vi "Multiple Chassis Synchronization - Scopes Synchronized without TCLK.vi"() -> ()   [LabVIEW 2026]
uses:
  SubVIs/NI SYNC Abstraction/Lib/Clock Routing.ctl
  <instrlib>/niScope/Controls/niScope export destinations.ctl
  SubVIs/NI SYNC Abstraction/Lib/Trigger Routing.ctl
  Types/State.WithoutTclk.ctl
  <instrlib>/niScope/Controls/niScope input clock source.ctl
  Types/MyVariables.ctl
  <instrlib>/niScope/Controls/niScope exportable signals.ctl
  <instrlib>/niFgen/niFgen.llb/niFgen Output Mode.ctl
  <instrlib>/niScope/Configure/Trigger/niScope Configure Trigger Edge.vi
  <instrlib>/niScope/Configure/Trigger/niScope Configure Trigger Digital.vi
  SubVIs/NI SYNC Abstraction/Lib/Connect Clock Terminals-Array.vi
  SubVIs/NI SYNC Abstraction/Lib/Connect Clock Terminals.vi
  SubVIs/NI SYNC Abstraction/Lib/Connect Trigger Terminals.vi
  <instrlib>/niScope/Acquire/Fetch/niScope Fetch Cluster.vi
  SubVIs/NI SYNC Abstraction/Lib/Disonnect Trigger Terminals.vi
  SubVIs/NI SYNC Abstraction/Lib/Disconnect Clock Terminals-Array.vi
  SubVIs/NI SYNC Abstraction/Lib/Disconnect Clock Terminals.vi
  <instrlib>/niSync/niSync.llb/niSync Initialize (IVI).vi
panel:
  in  "Tab Control":T1(tab)
  in  "Master.Scope":refnum<k15>="PXI1_SCOPE1"
  in  "Rest.Scopes":refnum<k15>[](array[refnum])=["PXI2_SCOPE2"]
  in  "Master.6674T_1":refnum<k15>="PXI1_MasterSync"
  in  "Rest.6674T_1":refnum<k15>="PXI2_SlaveSync"
  in  "FGEN.Ref":refnum<k15>="PXI1_FGEN1"
  in  "Routing":enum32{"Clock Routing", "Reference Trigger"}(tab)
  in  "Rest.In --> Clk10":T2={"Source Terminal"="ClkIn", "Destination Terminal"="PXI_Clk10_In"}
  in  "Master.In --> Clk10":T2={"Source Terminal"="ClkIn", "Destination Terminal"="PXI_Clk10_In"}
  in  "Master.Clock --> Out":T2={"Source Terminal"="Oscillator", "Destination Terminal"="ClkOut"}
  in  "Rest.Ref Trigger Source":T3="VAL_RTSI_0"
  in  "Rest.PFI --> Ref Trigger":T4={"Source"="PFI0", "Destination"="PXI_Trig0", "Synchronization Clock"="SyncClkAsync"}
  in  "Master.Ref Trigger --> PFI":T4={"Source"="PXI_Trig0", "Destination"="PFI0", "Synchronization Clock"="SyncClkAsync"}
  in  "Master.Ref Trigger Export":T3="VAL_RTSI_0"
  out "Waveform Graph":T5(graph)
  out "Sample Offset":dbl
  out "error out":errorcluster
  out "Offset Time (s)":dbl format="%#_p"
  # "Scope"
  # "Sync"
  # "Master"
  # "Ref Trigger Export"
  # "None"
  # "None"
  # "None"
  # "Sync"
  # "Scope"
  # "Rest"
  # "Ref Trigger Source"
  # "None"
  # "None"
  # "None"
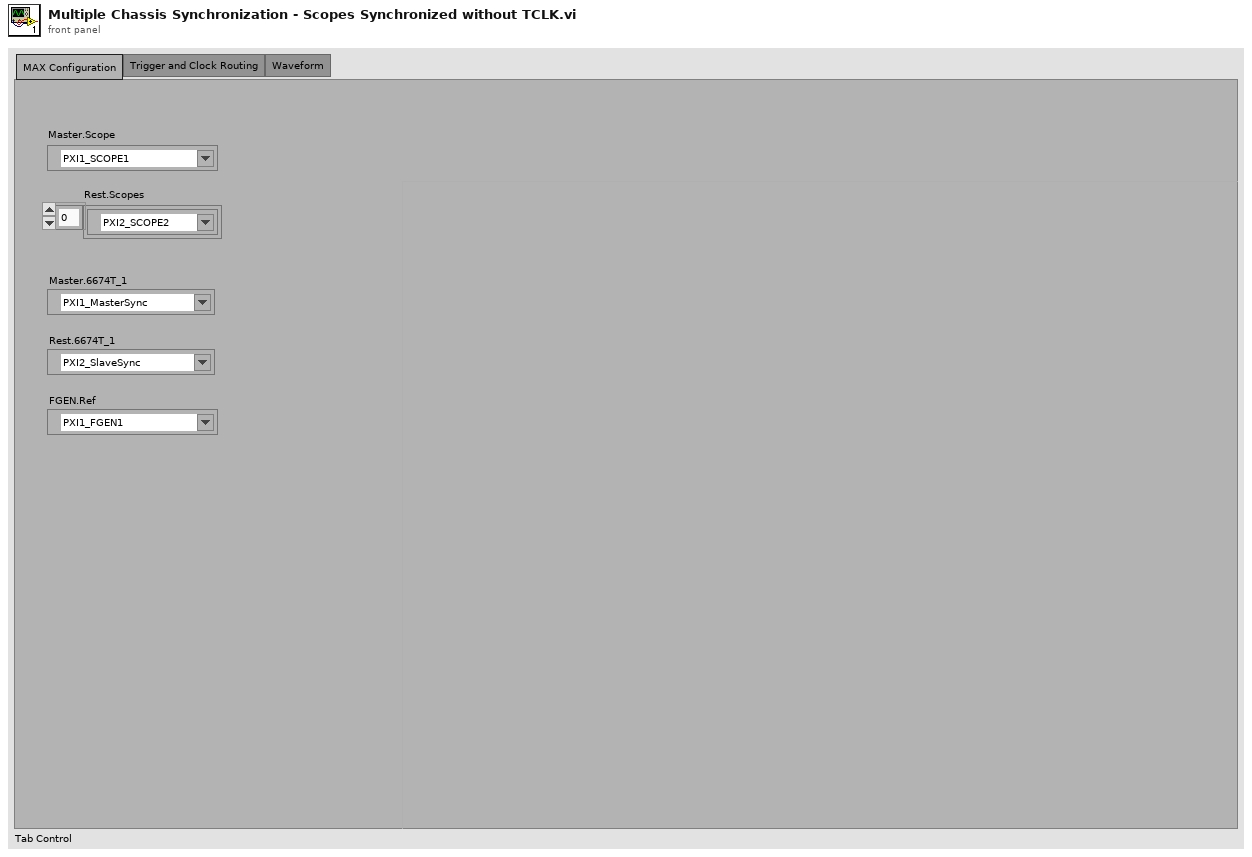
[diagram p1: front panel]
types:
  T1 = enum32{"MAX Configuration", "Trigger and Clock Routing", "Waveform"}
  T2 = typedef "Clock Routing.ctl" = cluster{"Source Terminal":string, "Destination Terminal":string}
  T3 = typedef "niScope export destinations.ctl" = string
  T4 = typedef "Trigger Routing.ctl" = cluster{"Source":string, "Destination":string, "Synchronization Clock":string}
  T5 = cluster{"relativeInitialX":dbl, "xIncrement":dbl, "wfm":dbl[]}[]
  T6 = typedef "niScope input clock source.ctl" = u16
  T7 = typedef "State.WithoutTclk.ctl" = enum16{"Initialize", "SCOPE: Config.Master", "SCOPE: Config.Rest", "SYNC: Device.Init", "SYNC: ConnectClock.Master", "SYNC: ConnectClock.Rest", "SYNC: ConnectRefTrigger.Master", "SYNC: ConnectRefTrigger.Rest", "SCOPE: Start", "FGEN: StartSquareWave", "SCOPE: Acquire", "FGEN: StopSquareWave", "SYNC: DisconnectRefTrigger.Master", "SYNC: DisconnectRefTrigger.Rest", "SYNC: DisconnectClock.Master", "SYNC: DisconnectClock.Rest", "Shutdown"}
  T8 = typedef "MyVariables.ctl" = cluster{"Master":cluster{"TimeSync.Ref":refnum<k15>, "TCLK.Ref":refnum<k20>, "Clock":cluster{"Clock --> Out":T2, "In --> Clk10":T2}, "Sync Pulse":cluster{"Sync Pulse Export":string, "Sync Pulse Export --> PFI":T4, "PFI --> Sync Pulse Source":T4, "Sync Pulse Source":string}, "Start Trigger":cluster{"Start Trigger Export":T3, "Start Trigger --> PFI":T4}, "Scope.Ref":refnum<k15>, "Ref Trigger":cluster{"Ref Trigger Export":T3, "Ref Trigger --> PFI":T4}}, "Rest":cluster{"TimeSync.Ref":refnum<k15>, "TCLK.Refs":refnum<k20>[], "Clock":cluster{"In --> Clk10":T2}, "Sync Pulse":cluster{"PFI --> Sync Pulse Source":T4, "Sync Pulse Source":string}, "Start Trigger":cluster{"PFI --> Start Trigger":T4, "Start Trigger Source":T3}, "Scope.Refs":refnum<k15>[], "Ref Trigger":cluster{"PFI --> Ref Trigger":T4, "Ref Trigger Source":T3}}, "FGEN.Ref":refnum<k15>}
  T9 = typedef "niScope exportable signals.ctl" = u16
  T10 = typedef "niFgen Output Mode.ctl" = u32
  T11 = cluster{"relativeInitialX":dbl, "xIncrement":dbl, "wfm":dbl[]}
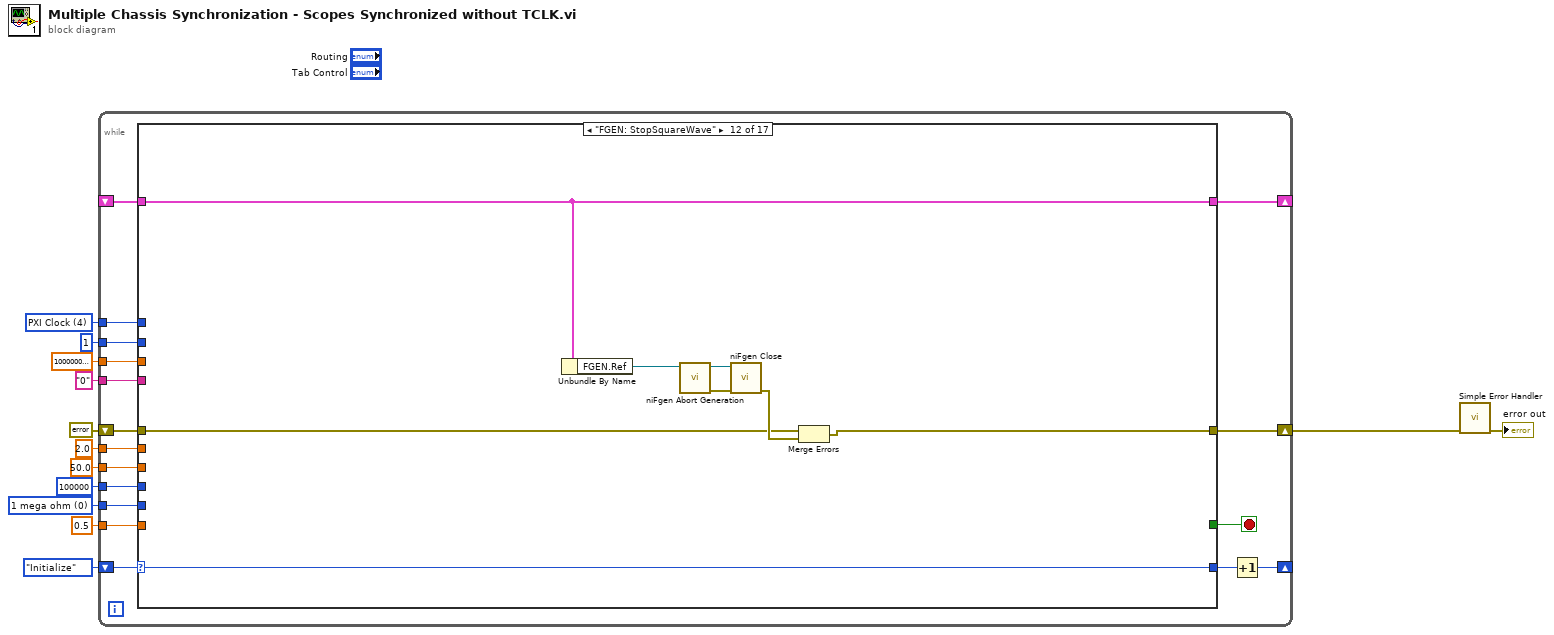
[diagram p0: block diagram]
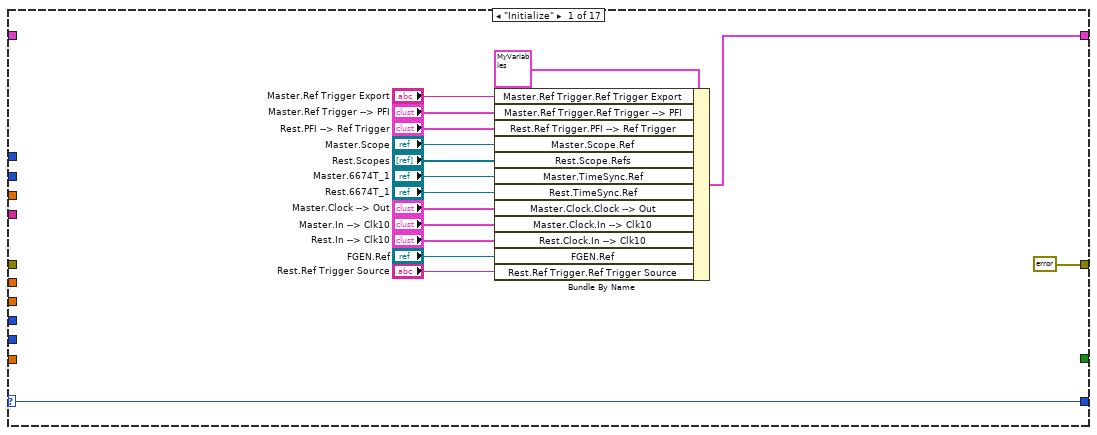
[diagram p2: hidden frame]
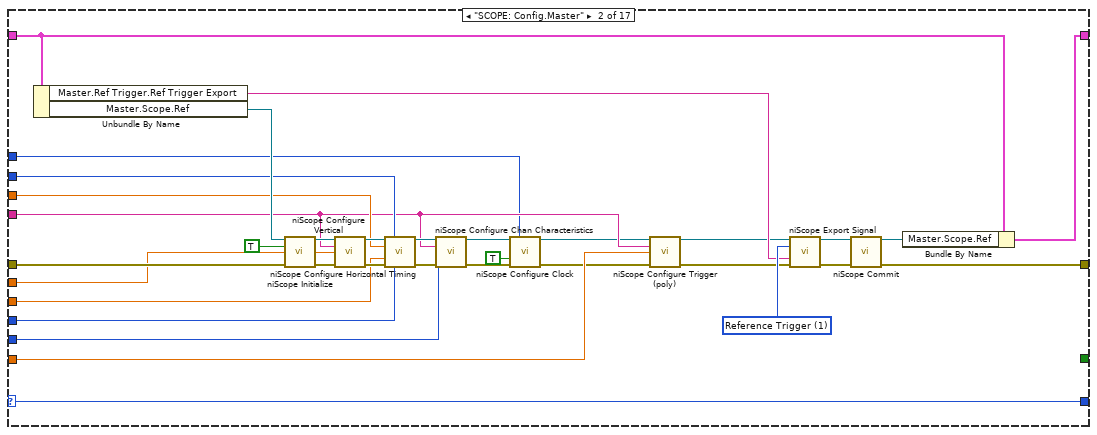
[diagram p3: hidden frame]
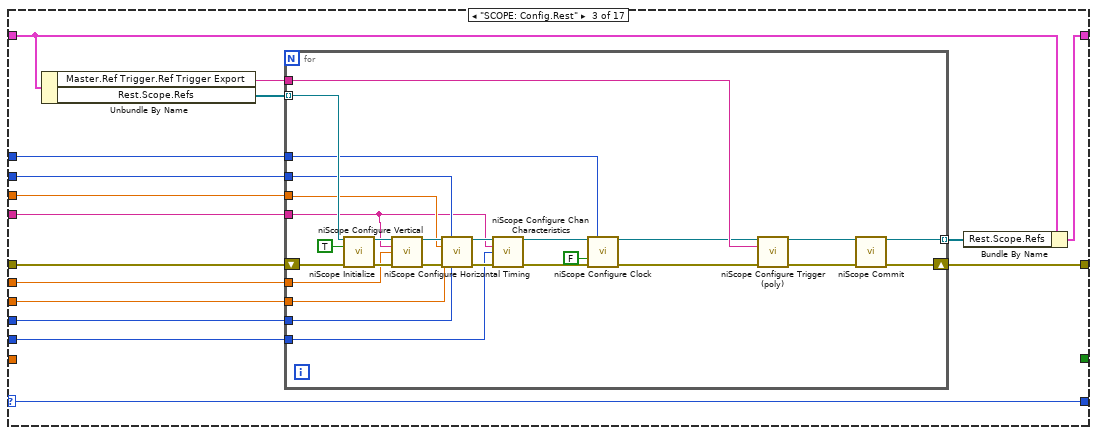
[diagram p4: hidden frame]
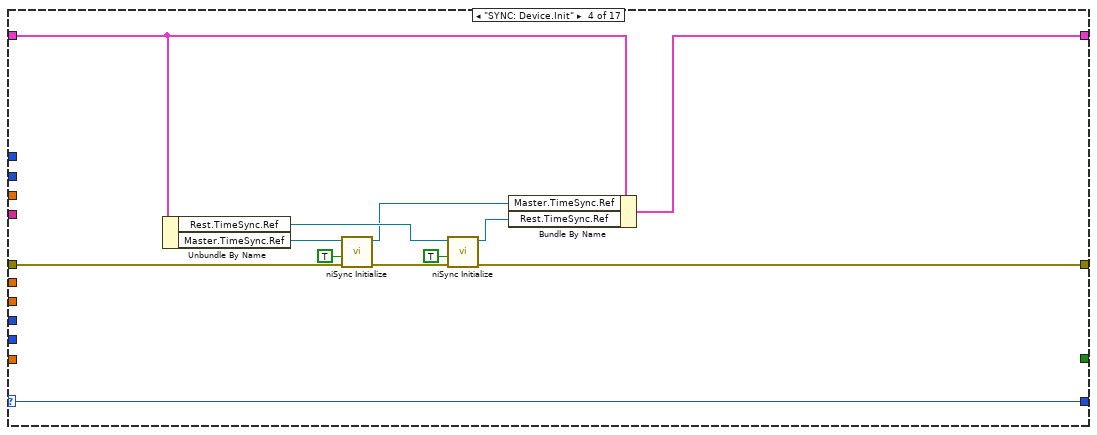
[diagram p5: hidden frame]
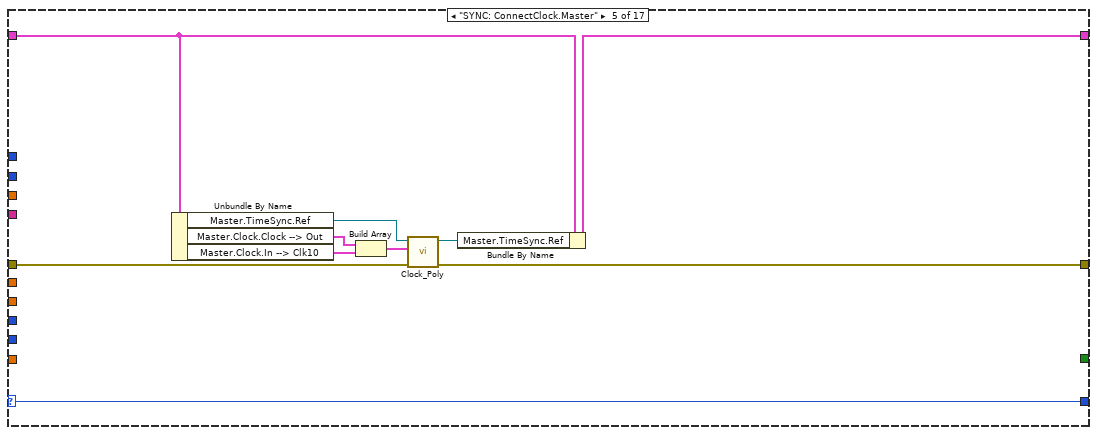
[diagram p6: hidden frame]
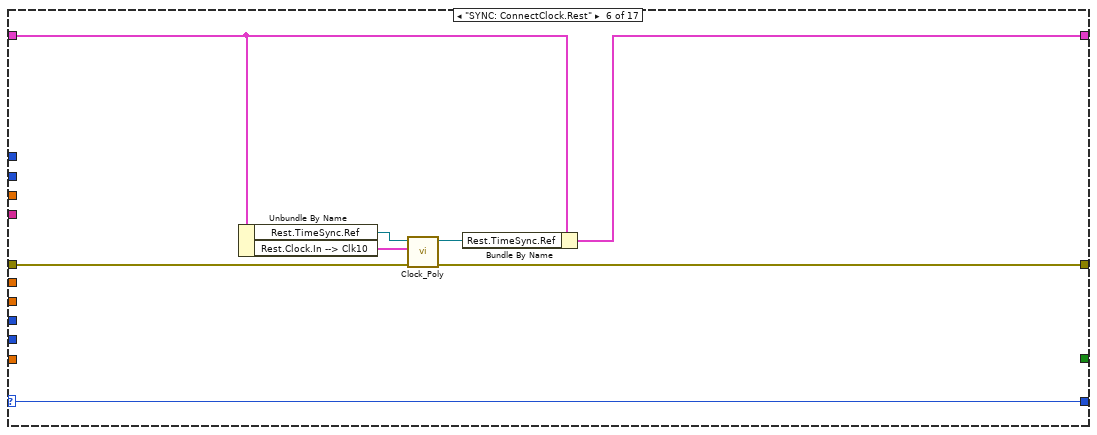
[diagram p7: hidden frame]
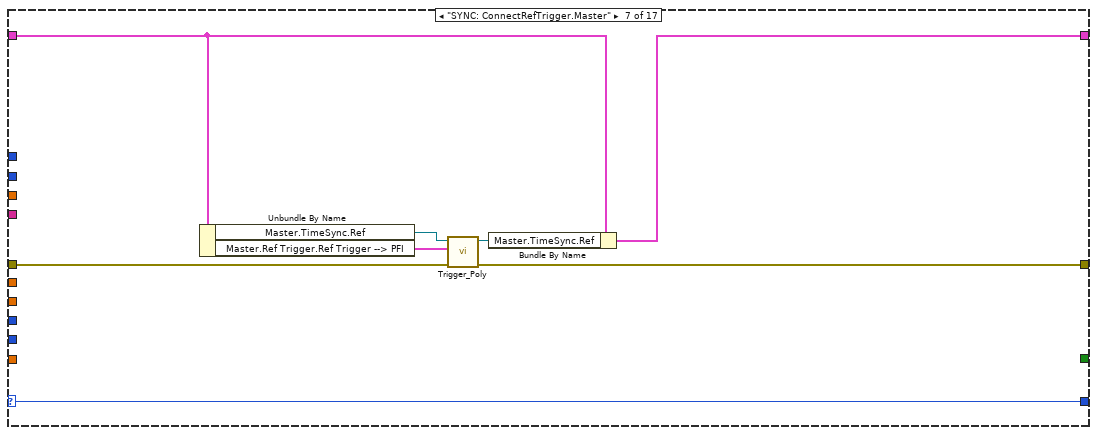
[diagram p8: hidden frame]
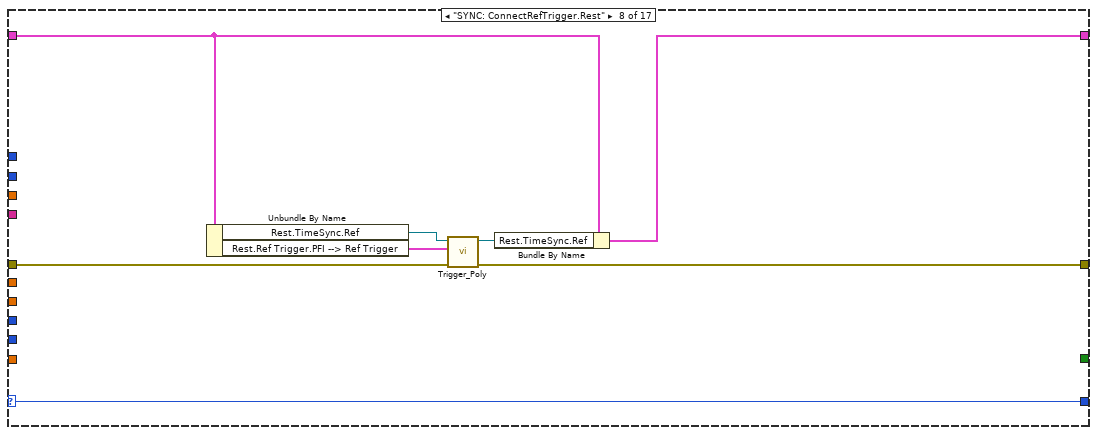
[diagram p9: hidden frame]
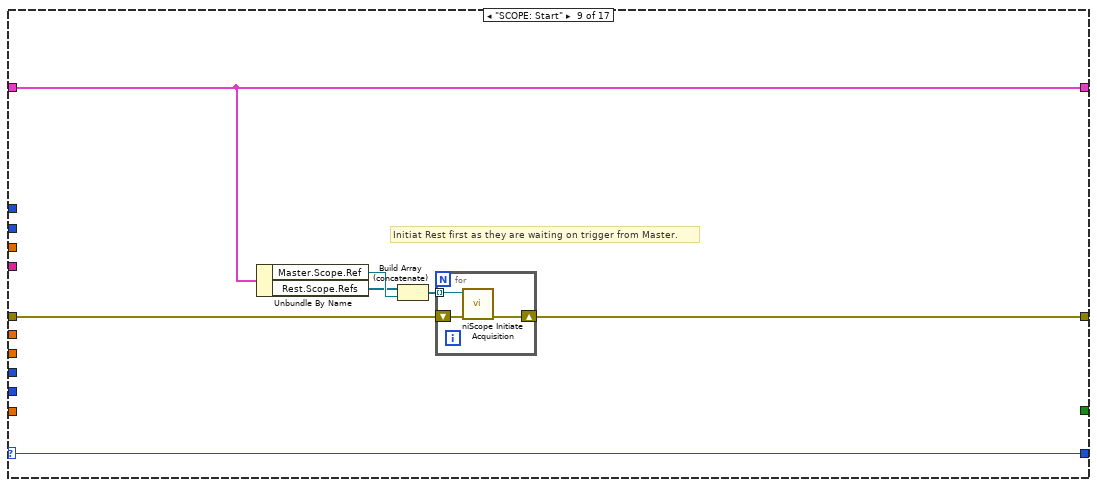
[diagram p10: hidden frame]
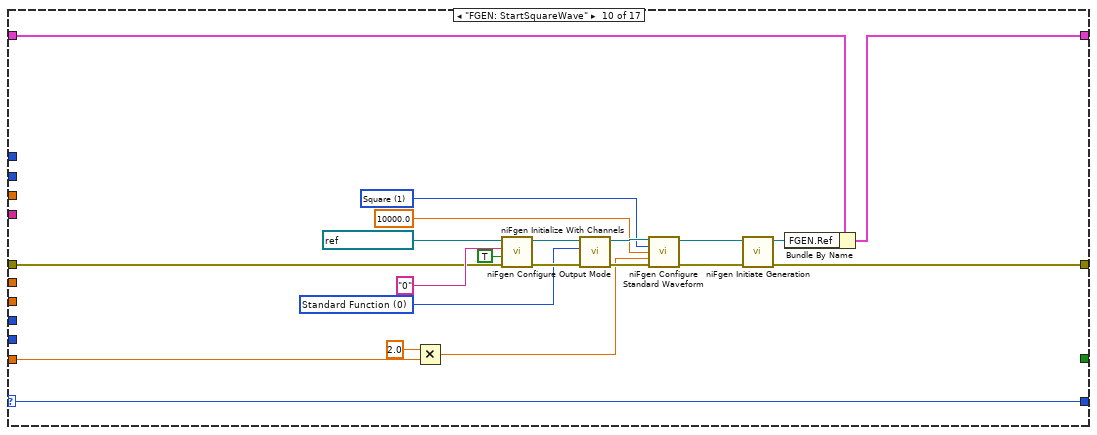
[diagram p11: hidden frame]
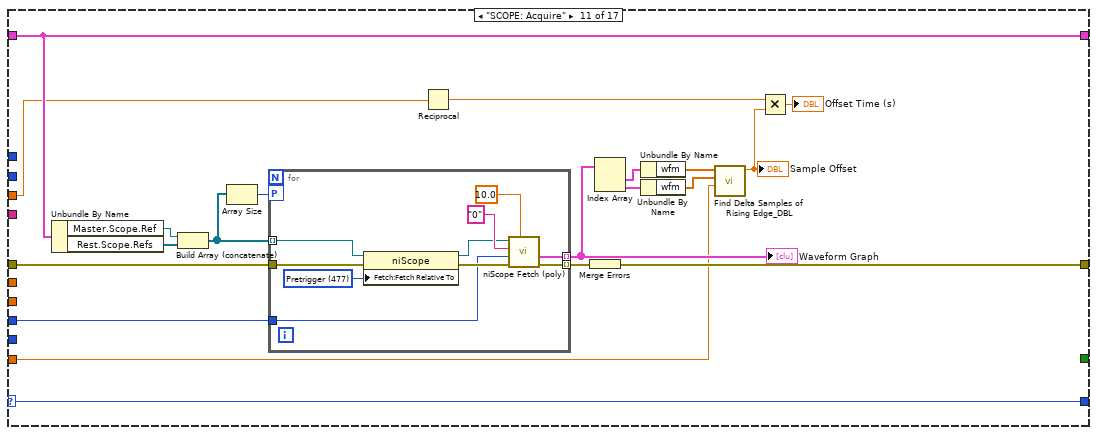
[diagram p12: hidden frame]
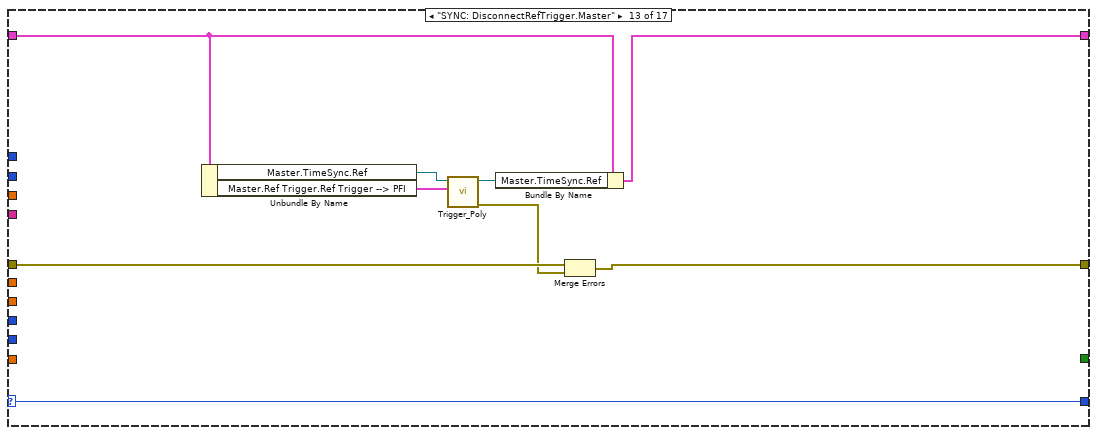
[diagram p13: hidden frame]
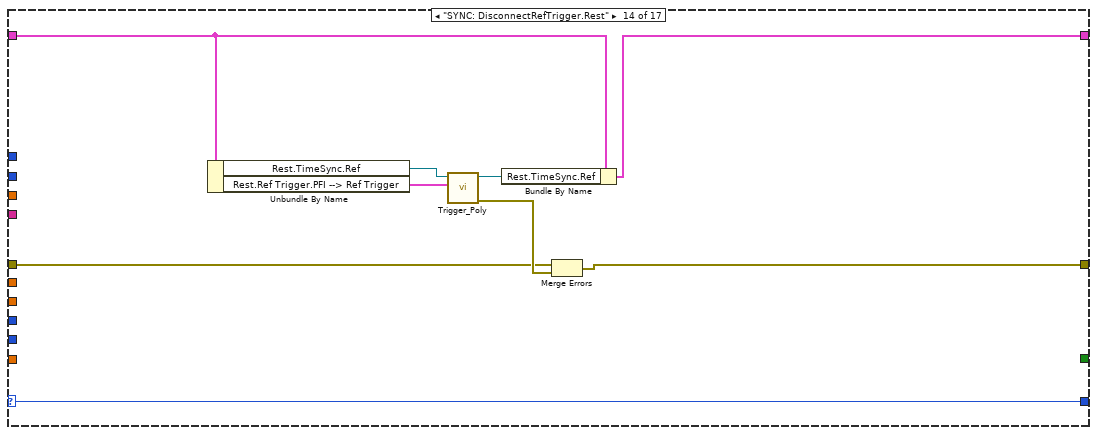
[diagram p14: hidden frame]
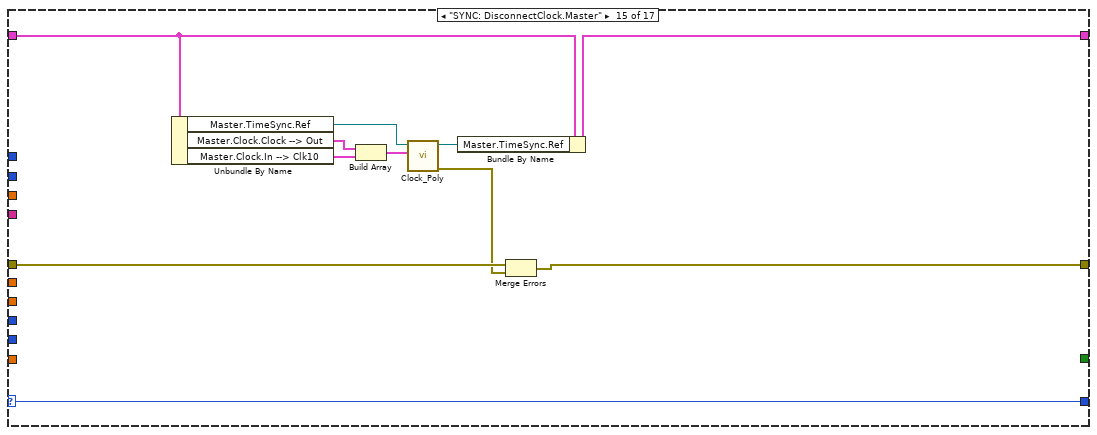
[diagram p15: hidden frame]
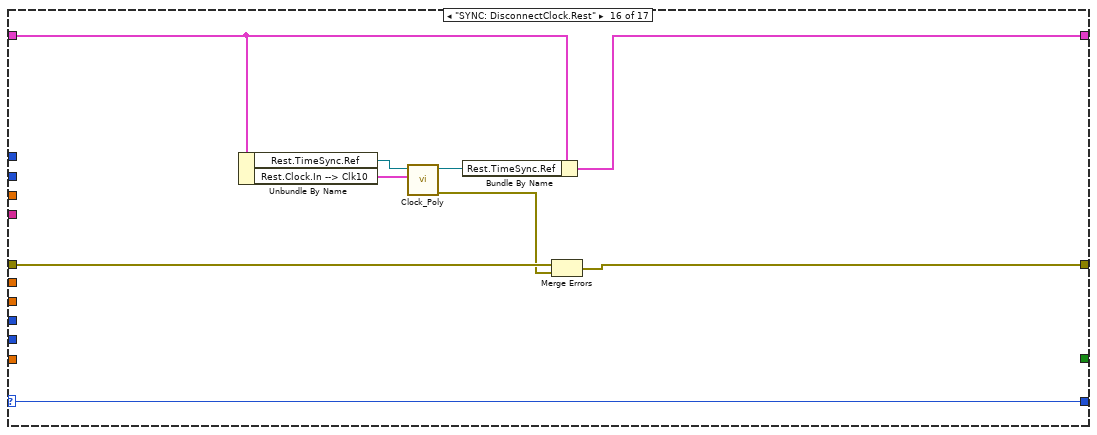
[diagram p16: hidden frame]
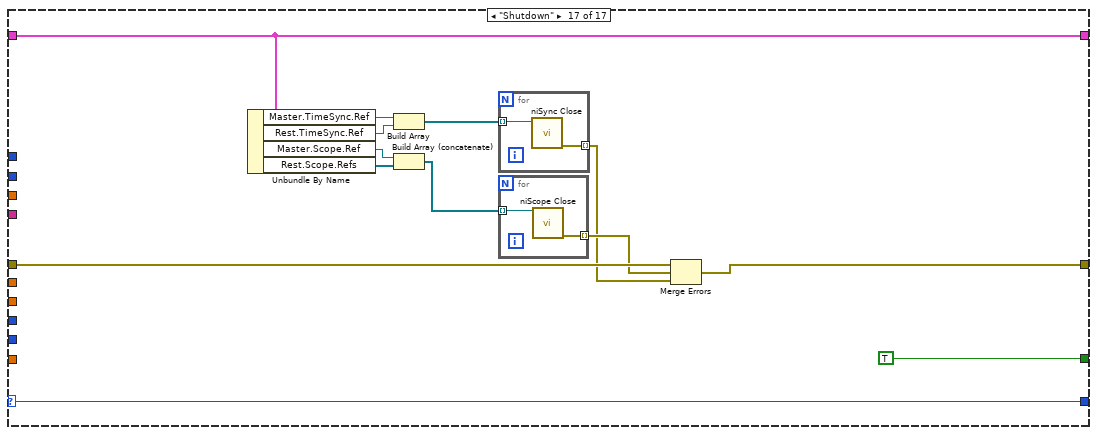
[diagram p17: hidden frame]
diagram:
  w1 = T6 4 items=["None"=0, "RTSI Clock"=1, "PFI 0"=6, "PFI 1"=2, "PFI 2"=3, "PXI Clock"=4, "External"=5, "Clock In"=7] ("input clock source")
  w5 = u32 0 items=["1 mega ohm"=0, "50 ohms"=2] ("input impedance")
  n1 = while {
    shift-right: [w23] -> _
    shift-left: State.WithoutTclk."Initialize" -> [w30]
    shift-right: [w29] -> _
    shift-left: _ -> [w28]
    shift-right: [w26] -> w11
    shift-left: errorcluster {"status"=FALSE, "code"=0, "source"=""} ("error out") -> [w27]
    tunnel: 100000000.0 ("min sample rate") -> [w22]
    tunnel: 100000 ("min record length") -> [w21]
    tunnel: 2.0 ("vertical offset") -> [w20]
    tunnel: 50.0 ("reference position") -> [w19]
    tunnel: w5 -> [w18]
    tunnel: 1 ("number of records") -> [w17]
    tunnel: "0" ("channels") -> [w16]
    tunnel: 0.5 ("trigger level") -> [w15]
    tunnel: w1 -> [w14]
    stop <- w24 stop-if-true
    n2 = case shown="\"FGEN: StopSquareWave\"" w30 {
      selector: w30 -> [w39 w80 w96 w125 w136 w147 w155 w163 w176 w187 w220 w231 w243 w252 w260 w272 w278]
      tunnel: [w40 w79 w95 w129 w144 w152 w160 w168 w173 w184 w217 w236 w246 w255 w266 w275 w289] -> w29
      tunnel: w28 -> [_ w70 w92 w130 w145 w153 w161 w169 w173 w186 w217 w236 w247 w256 w267 w276 w289]
      tunnel: [w39 w80 w96 w125 w136 w147 w155 w163 w176 w187 w220 w231 w243 w252 w260 w272 w278] -> w25
      tunnel: [errorcluster {"status"=FALSE, "code"=0, "source"=""} ("error out") w56 w94 w126 w141 w149 w157 w165 w171 w188 w214 w232 w239 w249 w258 w269 w279] -> w26
      tunnel: w27 -> [_ w71 w93 w124 w137 w148 w156 w164 w172 w189 w219 w233 w241 w248 w259 w270 w282]
      tunnel: [_ _ _ _ _ _ _ _ _ _ _ _ _ _ _ _ TRUE] -> w24
      tunnel: w22 -> [_ w64 w87 _ _ _ _ _ _ _ w205 _ _ _ _ _ _]
      tunnel: w21 -> [_ w63 w83 _ _ _ _ _ _ _ w206 _ _ _ _ _ _]
      tunnel: w20 -> [_ w62 w85 _ _ _ _ _ _ _ _ _ _ _ _ _ _]
      tunnel: w19 -> [_ w61 w84 _ _ _ _ _ _ _ _ _ _ _ _ _ _]
      tunnel: w18 -> [_ w60 w82 _ _ _ _ _ _ _ _ _ _ _ _ _ _]
      tunnel: w17 -> [_ w59 w88 _ _ _ _ _ _ _ _ _ _ _ _ _ _]
      tunnel: w16 -> [_ w58 w86 _ _ _ _ _ _ _ _ _ _ _ _ _ _]
      tunnel: w15 -> [_ w57 _ _ _ _ _ _ _ w182 w201 _ _ _ _ _ _]
      tunnel: w14 -> [_ w47 w81 _ _ _ _ _ _ _ _ _ _ _ _ _ _]
      frame "Initialize" {
        n3 = Bundle By Name(cluster=T8 {"Master"={"TimeSync.Ref"="PXI_Trig0", "TCLK.Ref"=refnum, "Clock"={"Clock --> Out"={"Source Terminal"="Oscillator", "Destination Terminal"="ClkOut"}, "In --> Clk10"={"Source Terminal"="ClkIn", "Destination Terminal"="PXI_Clk10_In"}}, "Sync Pulse"={"Sync Pulse Export"="SyncClkFullSpeed", "Sync Pulse Export --> PFI"={"Source"="ClkIn", "Destination"="PXI_Clk10_In", "Synchronization Clock"="SyncClkAsync"}, "PFI --> Sync Pulse Source"={"Source"="PXI_Trig2", "Destination"="PFI2", "Synchronization Clock"="SyncClkAsync"}, "Sync Pulse Source"="PFI1"}, "Start Trigger"={"Start Trigger Export"="PXI_Trig2", "Start Trigger --> PFI"={"Source"="SyncClkAsync", "Destination"="VAL_RTSI_2", "Synchronization Clock"=""}}, "Scope.Ref"="", "Ref Trigger"={"Ref Trigger Export"="VAL_RTSI_2", "Ref Trigger --> PFI"={"Source"="PXI_Trig3", "Destination"="PFI0", "Synchronization Clock"="SyncClkAsync"}}}, "Rest"={"TimeSync.Ref"="", "TCLK.Refs"=[], "Clock"={"In --> Clk10"={"Source Terminal"="PXI_Trig0", "Destination Terminal"="PFI2"}}, "Sync Pulse"={"PFI --> Sync Pulse Source"={"Source"="PFI1", "Destination"="PXI_Trig1", "Synchronization Clock"="SyncClkAsync"}, "Sync Pulse Source"="PXI_Trig1"}, "Start Trigger"={"PFI --> Start Trigger"={"Source"="PFI1", "Destination"="PXI_Trig2", "Synchronization Clock"="SyncClkAsync"}, "Start Trigger Source"="VAL_RTSI_2"}, "Scope.Refs"=[], "Ref Trigger"={"PFI --> Ref Trigger"={"Source"="PFI0", "Destination"="PXI_Trig3", "Synchronization Clock"="SyncClkAsync"}, "Ref Trigger Source"="VAL_RTSI_3"}}, "FGEN.Ref"=""} ("Routes"), "Master.Ref Trigger.Ref Trigger Export"="Master.Ref Trigger Export", "Master.Ref Trigger.Ref Trigger --> PFI"="Master.Ref Trigger --> PFI", "Rest.Ref Trigger.PFI --> Ref Trigger"="Rest.PFI --> Ref Trigger", "Master.Scope.Ref"="Master.Scope", "Rest.Scope.Refs"="Rest.Scopes", "Master.TimeSync.Ref"="Master.6674T_1", "Rest.TimeSync.Ref"="Rest.6674T_1", "Master.Clock.Clock --> Out"="Master.Clock --> Out", "Master.Clock.In --> Clk10"="Master.In --> Clk10", "Rest.Clock.In --> Clk10"="Rest.In --> Clk10", "FGEN.Ref"="FGEN.Ref", "Rest.Ref Trigger.Ref Trigger Source"="Rest.Ref Trigger Source") -> (w40:T8)
      }
      frame "SCOPE: Config.Master" {
        w66 = T9 1 items=["None"=0, "Start Trigger"=2, "Advance Trigger"=5, "Reference Trigger"=1, "End of Record Event"=4, "End of Acquisition Event"=3, "Ready for Start Event"=7, "Ready for Advance Event"=6, "Ready for Reference Event"=10, "Reference Clock"=100, "Sample Clock"=101, "5 Volt Power"=13] ("signal")
        n4 = Unbundle By Name(w70) -> ("Master.Ref Trigger.Ref Trigger Export"=w65:T3, "Master.Scope.Ref"=w69:refnum<k15>)
        n5 = call <instrlib>:"niScope Initialize.vi"("resource name"=w69, "id query"=TRUE, "error in"=w71) -> ("instrument handle"=w77:refnum<k15>, "error out"=w74:errorcluster)  [unwired: 11 in]
        n6 = call <instrlib>:"niScope Configure Vertical.vi"("instrument handle"=w77, "channels"=w58, "vertical range"=w62, "error in"=w74) -> ("instrument handle out"=w76:refnum<k15>, "error out"=w73:errorcluster)  [unwired: 10 in]
        n7 = call <instrlib>:"niScope Configure Horizontal Timing.vi"("instrument handle"=w76, "number of records"=w59, "min sample rate"=w64, "reference position"=w61, "error in"=w73, "min record length"=w63) -> ("instrument handle out"=w75:refnum<k15>, "error out"=w72:errorcluster)  [unwired: 8 in]
        n8 = call <instrlib>:"niScope Configure Chan Characteristics.vi"("instrument handle"=w75, "channels"=w58, "input impedance"=w60, "error in"=w72) -> ("instrument handle out"=w49:refnum<k15>, "error out"=w51:errorcluster)  [unwired: 10 in]
        n9 = call <instrlib>:"niScope Configure Clock.vi"("instrument handle"=w49, "input clock source"=w47, "master enabled"=TRUE, "error in"=w51) -> ("instrument handle out"=w48:refnum<k15>, "error out"=w50:errorcluster)  [unwired: 10 in]
        n10 = call-poly <instrlib>:"niScope Configure Trigger (poly).vi"("instrument handle"=w48, "trigger source"=w58, "trigger level"=w57, "error in"=w50) -> ("instrument handle out"=w53:refnum<k15>, "error out"=w54:errorcluster)  [unwired: 10 in]
        n11 = call <instrlib>:"niScope Export Signal.vi"("instrument handle"=w53, "signal"=w66, "output terminal"=w65, "error in"=w54) -> ("instrument handle out"=w67:refnum<k15>, "error out"=w68:errorcluster)  [unwired: 10 in]
        n12 = call <instrlib>:"niScope Commit.vi"("instrument handle"=w67, "error in"=w68) -> ("instrument handle out"=w55:refnum<k15>, "error out"=w56:errorcluster)  [unwired: 12 in]
        n13 = Bundle By Name(cluster=w70, "Master.Scope.Ref"=w55) -> (w79:T8)
      }
      frame "SCOPE: Config.Rest" {
        n14 = Unbundle By Name(w92) -> ("Master.Ref Trigger.Ref Trigger Export"=w89:T3, "Rest.Scope.Refs"=w90:refnum<k15>[])
        n15 = for {
          shift-right: [w104] -> w94
          shift-left: w93 -> [w116]
          tunnel: [w103] -> w91 mode=indexing
          tunnel: w90 -> [w113] mode=indexing
          tunnel: w89 -> [w112]
          tunnel: w88 -> [w111]
          tunnel: w87 -> [w110]
          tunnel: w86 -> [w109]
          tunnel: w85 -> [w108]
          tunnel: w84 -> [w107]
          tunnel: w83 -> [w106]
          tunnel: w82 -> [w105]
          tunnel: w81 -> [w97]
          n16 = call <instrlib>:"niScope Initialize.vi"("resource name"=w113, "id query"=TRUE, "error in"=w116) -> ("instrument handle"=w122:refnum<k15>, "error out"=w119:errorcluster)  [unwired: 11 in]
          n17 = call <instrlib>:"niScope Configure Vertical.vi"("instrument handle"=w122, "channels"=w109, "vertical range"=w108, "error in"=w119) -> ("instrument handle out"=w121:refnum<k15>, "error out"=w118:errorcluster)  [unwired: 10 in]
          n18 = call <instrlib>:"niScope Configure Horizontal Timing.vi"("instrument handle"=w121, "number of records"=w111, "min sample rate"=w110, "reference position"=w107, "error in"=w118, "min record length"=w106) -> ("instrument handle out"=w120:refnum<k15>, "error out"=w117:errorcluster)  [unwired: 8 in]
          n19 = call <instrlib>:"niScope Configure Chan Characteristics.vi"("instrument handle"=w120, "channels"=w109, "input impedance"=w105, "error in"=w117) -> ("instrument handle out"=w101:refnum<k15>, "error out"=w99:errorcluster)  [unwired: 10 in]
          n20 = call <instrlib>:"niScope Configure Clock.vi"("instrument handle"=w101, "input clock source"=w97, "master enabled"=FALSE, "error in"=w99) -> ("instrument handle out"=w100:refnum<k15>, "error out"=w98:errorcluster)  [unwired: 10 in]
          n21 = call-poly <instrlib>:"niScope Configure Trigger (poly).vi"("instrument handle"=w100, "trigger source"=w112, "error in"=w98) -> ("instrument handle out"=w114:refnum<k15>, "error out"=w115:errorcluster)  [unwired: 11 in]
          n22 = call <instrlib>:"niScope Commit.vi"("instrument handle"=w114, "error in"=w115) -> ("instrument handle out"=w103:refnum<k15>, "error out"=w104:errorcluster)  [unwired: 12 in]
        }
        n23 = Bundle By Name(cluster=w92, "Rest.Scope.Refs"=w91) -> (w95:T8)
      }
      frame "SYNC: Device.Init" {
        n24 = Unbundle By Name(w130) -> ("Rest.TimeSync.Ref"=w134:refnum<k15>, "Master.TimeSync.Ref"=w135:refnum<k15>)
        n25 = call-poly <instrlib>:"niSync Initialize.vi"("error in (no error)"=w124, "reset device (F)"=TRUE, "resource name"=w135) -> ("error out"=w133:errorcluster, "instrument handle out"=w128:refnum<k15>)  [unwired: 7 in]
        n26 = call-poly <instrlib>:"niSync Initialize.vi"("error in (no error)"=w133, "reset device (F)"=TRUE, "resource name"=w134) -> ("error out"=w126:errorcluster, "instrument handle out"=w127:refnum<k15>)  [unwired: 7 in]
        n27 = Bundle By Name(cluster=w130, "Master.TimeSync.Ref"=w128, "Rest.TimeSync.Ref"=w127) -> (w129:T8)
      }
      frame "SYNC: ConnectClock.Master" {
        n28 = Unbundle By Name(w145) -> ("Master.TimeSync.Ref"=w143:refnum<k15>, "Master.Clock.Clock --> Out"=w140:T2, "Master.Clock.In --> Clk10"=w139:T2)
        n29 = Build Array(w140, w139) -> (w138:T2[])
        n30 = call-poly "Clock_Poly.vi"("error in (no error)"=w137, "Clock Routing"=w138, "instrument handle"=w143) -> ("error out"=w141:errorcluster, "instrument handle out"=w142:refnum<k15>)  [unwired: 7 in]
        n31 = Bundle By Name(cluster=w145, "Master.TimeSync.Ref"=w142) -> (w144:T8)
      }
      frame "SYNC: ConnectClock.Rest" {
        n32 = Unbundle By Name(w153) -> ("Rest.TimeSync.Ref"=w151:refnum<k15>, "Rest.Clock.In --> Clk10"=w146:T2)
        n33 = call-poly "Clock_Poly.vi"("error in (no error)"=w148, "Clock Routing"=w146, "instrument handle"=w151) -> ("error out"=w149:errorcluster, "instrument handle out"=w150:refnum<k15>)  [unwired: 7 in]
        n34 = Bundle By Name(cluster=w153, "Rest.TimeSync.Ref"=w150) -> (w152:T8)
      }
      frame "SYNC: ConnectRefTrigger.Master" {
        n35 = Unbundle By Name(w161) -> ("Master.TimeSync.Ref"=w159:refnum<k15>, "Master.Ref Trigger.Ref Trigger --> PFI"=w154:T4)
        n36 = call-poly "Trigger_Poly.vi"("error in (no error)"=w156, "Routing Information"=w154, "instrument handle"=w159) -> ("error out"=w157:errorcluster, "instrument handle out"=w158:refnum<k15>)  [unwired: 7 in]
        n37 = Bundle By Name(cluster=w161, "Master.TimeSync.Ref"=w158) -> (w160:T8)
      }
      frame "SYNC: ConnectRefTrigger.Rest" {
        n38 = Unbundle By Name(w169) -> ("Rest.TimeSync.Ref"=w167:refnum<k15>, "Rest.Ref Trigger.PFI --> Ref Trigger"=w162:T4)
        n39 = call-poly "Trigger_Poly.vi"("error in (no error)"=w164, "Routing Information"=w162, "instrument handle"=w167) -> ("error out"=w165:errorcluster, "instrument handle out"=w166:refnum<k15>)  [unwired: 7 in]
        n40 = Bundle By Name(cluster=w169, "Rest.TimeSync.Ref"=w166) -> (w168:T8)
      }
      frame "SCOPE: Start" {
        # "Initiat Rest first as they are waiting on trigger from Master."
        n41 = Unbundle By Name(w173) -> ("Master.Scope.Ref"=w175:refnum<k15>, "Rest.Scope.Refs"=w174:refnum<k15>[])
        n42 = Build Array (concatenate)(w174, w175) -> (w170:refnum<k15>[])
        n43 = for {
          shift-right: [w178] -> w171
          shift-left: w172 -> [w179]
          tunnel: w170 -> [w177] mode=indexing
          n44 = call <instrlib>:"niScope Initiate Acquisition.vi"("instrument handle"=w177, "error in"=w179) -> ("error out"=w178:errorcluster)  [unwired: 12 in, 1 out]
        }
      }
      frame "FGEN: StartSquareWave" {
        w192 = u16 1 items=["Sine", "Square", "Triangle", "Ramp Up", "Ramp Down", "DC", "Noise"] ("Standard Waveform")
        w190 = T10 0 items=["Standard Function", "Frequency List", "Arbitrary Waveform", "Arbitrary Sequence", "Script"] ("output mode")
        n45 = Multiply(x=2.0, y=w182) -> (x*y=w181:dbl)
        n46 = call <instrlib>:"niFgen Initialize With Channels.vi"("error in (no error)"=w189, "Reset Device (default: False)"=TRUE, "Channel Name"="0", "Resource Name"=refnum<k15> "PXI1_FGEN1" ("FGEN Resource Name")) -> ("error out"=w200:errorcluster, "Instrument Handle Out"=w199:refnum<k15>)  [unwired: 6 in]
        n47 = call <instrlib>:"niFgen Configure Output Mode.vi"("error in (no error)"=w200, "Output Mode (default: 0=Standard Function)"=w190, "Instrument Handle"=w199) -> ("error out"=w198:errorcluster, "Instrument Handle Out"=w197:refnum<k15>)  [unwired: 6 in]
        n48 = call <instrlib>:"niFgen Configure Standard Waveform.vi"("Instrument Handle"=w197, "Waveform"=w192, "Frequency"=10000.0, "Amplitude"=w181, "error in (no error)"=w198) -> ("Instrument Handle Out"=w196:refnum<k15>, "error out"=w195:errorcluster)  [unwired: 9 in]
        n49 = call <instrlib>:"niFgen Initiate Generation.vi"("error in (no error)"=w195, "Instrument Handle"=w196) -> ("error out"=w188:errorcluster, "Instrument Handle Out"=w185:refnum<k15>)  [unwired: 8 in]
        n50 = Bundle By Name(cluster=w186, "FGEN.Ref"=w185) -> (w184:T8)
      }
      frame "SCOPE: Acquire" {
        n51 = Unbundle By Name(w217) -> ("Master.Scope.Ref"=w215:refnum<k15>, "Rest.Scope.Refs"=w216:refnum<k15>[])
        n52 = Build Array (concatenate)(w215, w216) -> (w213:refnum<k15>[])
        n53 = Array Size(array=w213) -> (size(s)=w212:i32)
        n54 = for {
          tunnel: w213 -> [w227] mode=indexing
          tunnel: [w222] -> w207 mode=indexing
          tunnel: w219 -> [w226]
          tunnel: [w230] -> w218 mode=indexing
          workers-P: w212 -> [_]
          tunnel: w206 -> [w221]
          w223 = 477 items=["Start"=482, "Trigger"=483, "Pretrigger"=477, "Now"=481, "Read Pointer"=388] ("Fetch:Fetch Relative To")
          n55 = property class="niScope"(reference=w227, error in=w226, "Fetch:Fetch Relative To"=w223) -> (reference out=w224:refnum<k15>, error out=w225:errorcluster)
          n56 = call-poly <instrlib>:"niScope Fetch (poly).vi"("timeout"=10.0, "error in"=w225, "numSamples"=w221, "channels"="0", "instrument handle"=w224) -> ("error out"=w230:errorcluster, "waveform"=w222:T11)  [unwired: 3 in, 2 out]
        }
        "Waveform Graph" <- w207
        n57 = Reciprocal(x=w205) -> (1/x=w203:dbl)
        n58 = Merge Errors(w218) -> (w214:errorcluster)
        n59 = Index Array(array=w207) -> (element #1=w211:T11, element #2=w210:T11)  [unwired: 2 in]
        n60 = Unbundle By Name(w211) -> ("wfm"=w208:dbl[])
        n61 = Unbundle By Name(w210) -> ("wfm"=w209:dbl[])
        n62 = call "Find Delta Samples of Rising Edge_DBL.vi"("Trigger Level"=w201, "Channel 2"=w209, "Channel 1"=w208) -> ("Sample Offset"=w204:dbl)  [unwired: 8 in]
        "Sample Offset" <- w204
        n63 = Multiply(x=w203, y=w204) -> (x*y=→"Offset Time (s)":dbl)
      }
      frame "FGEN: StopSquareWave" {
        n64 = Unbundle By Name(w236) -> ("FGEN.Ref"=w235:refnum<k15>)
        n65 = call <instrlib>:"niFgen Abort Generation.vi"("Instrument Handle"=w235) -> ("error out"=w238:errorcluster, "Instrument Handle Out"=w237:refnum<k15>)  [unwired: 9 in]
        n66 = call <instrlib>:"niFgen Close.vi"("error in (no error)"=w238, "Instrument Handle"=w237) -> ("error out"=w234:errorcluster)  [unwired: 9 in]
        n67 = Merge Errors(w233, w234) -> (w232:errorcluster)
      }
      frame "SYNC: DisconnectRefTrigger.Master" {
        n68 = Unbundle By Name(w247) -> ("Master.TimeSync.Ref"=w245:refnum<k15>, "Master.Ref Trigger.Ref Trigger --> PFI"=w242:T4)
        n69 = call-poly "Trigger_Poly.vi"("Routing Information"=w242, "instrument handle"=w245) -> ("error out"=w240:errorcluster, "instrument handle out"=w244:refnum<k15>)  [unwired: 8 in]
        n70 = Bundle By Name(cluster=w247, "Master.TimeSync.Ref"=w244) -> (w246:T8)
        n71 = Merge Errors(w241, w240) -> (w239:errorcluster)
      }
      frame "SYNC: DisconnectRefTrigger.Rest" {
        n72 = Unbundle By Name(w256) -> ("Rest.TimeSync.Ref"=w254:refnum<k15>, "Rest.Ref Trigger.PFI --> Ref Trigger"=w251:T4)
        n73 = call-poly "Trigger_Poly.vi"("Routing Information"=w251, "instrument handle"=w254) -> ("error out"=w250:errorcluster, "instrument handle out"=w253:refnum<k15>)  [unwired: 8 in]
        n74 = Bundle By Name(cluster=w256, "Rest.TimeSync.Ref"=w253) -> (w255:T8)
        n75 = Merge Errors(w248, w250) -> (w249:errorcluster)
      }
      frame "SYNC: DisconnectClock.Master" {
        n76 = Unbundle By Name(w267) -> ("Master.TimeSync.Ref"=w265:refnum<k15>, "Master.Clock.Clock --> Out"=w263:T2, "Master.Clock.In --> Clk10"=w262:T2)
        n77 = Build Array(w263, w262) -> (w261:T2[])
        n78 = call-poly "Clock_Poly.vi"("Clock Routing"=w261, "instrument handle"=w265) -> ("error out"=w257:errorcluster, "instrument handle out"=w264:refnum<k15>)  [unwired: 8 in]
        n79 = Bundle By Name(cluster=w267, "Master.TimeSync.Ref"=w264) -> (w266:T8)
        n80 = Merge Errors(w259, w257) -> (w258:errorcluster)
      }
      frame "SYNC: DisconnectClock.Rest" {
        n81 = Unbundle By Name(w276) -> ("Rest.TimeSync.Ref"=w274:refnum<k15>, "Rest.Clock.In --> Clk10"=w271:T2)
        n82 = call-poly "Clock_Poly.vi"("Clock Routing"=w271, "instrument handle"=w274) -> ("error out"=w268:errorcluster, "instrument handle out"=w273:refnum<k15>)  [unwired: 8 in]
        n83 = Bundle By Name(cluster=w276, "Rest.TimeSync.Ref"=w273) -> (w275:T8)
        n84 = Merge Errors(w270, w268) -> (w269:errorcluster)
      }
      frame "Shutdown" {
        n85 = Unbundle By Name(w289) -> ("Master.TimeSync.Ref"=w288:refnum<k15>, "Rest.TimeSync.Ref"=w287:refnum<k15>, "Master.Scope.Ref"=w286:refnum<k15>, "Rest.Scope.Refs"=w285:refnum<k15>[])
        n86 = Build Array(w288, w287) -> (w283:refnum<k15>[])
        n87 = Build Array (concatenate)(w286, w285) -> (w284:refnum<k15>[])
        n88 = for {
          tunnel: w283 -> [w291] mode=indexing
          tunnel: [w290] -> w280 mode=indexing
          n89 = call <instrlib>:"niSync Close.vi"("instrument handle"=w291) -> ("error out"=w290:errorcluster)  [unwired: 10 in]
        }
        n90 = for {
          tunnel: w284 -> [w293] mode=indexing
          tunnel: [w292] -> w281 mode=indexing
          n91 = call <instrlib>:"niScope Close.vi"("instrument handle"=w293) -> ("error out"=w292:errorcluster)  [unwired: 14 in]
        }
        n92 = Merge Errors(w282, w281, w280) -> (w279:errorcluster)
      }
    }
    n93 = Increment(x=w25) -> (x+1=w23:T7)
  }
  n94 = call <vilib>:"Simple Error Handler.vi"("error in (no error)"=w11) -> ("error out"=→"error out":errorcluster)  [unwired: 4 in, 4 out]
